vi "PeriodicTaskMatrix.vi"(8 "Error In":errorcluster, 9 "Smart Write (T)?":bool=TRUE, 10 "LEDs to Light":bool[][](array[boolean])=[[TRUE, TRUE, TRUE, TRUE, TRUE, TRUE, TRUE, FALSE], [TRUE, TRUE, TRUE, TRUE, TRUE, TRUE, FALSE, FALSE], [TRUE, TRUE, TRUE, TRUE, TRUE, FALSE, FALSE, FALSE], [TRUE, TRUE, TRUE, TRUE, FALSE, FALSE, FALSE, FALSE], [TRUE, TRUE, TRUE, FALSE, FALSE, FALSE, FALSE, FALSE], [TRUE, TRUE, FALSE, FALSE, FALSE, FALSE, FALSE, FALSE], [TRUE, FALSE, FALSE, FALSE, FALSE, FALSE, FALSE, FALSE], [FALSE, FALSE, FALSE, FALSE, FALSE, FALSE, FALSE, TRUE]], 11 "LINX Resource":T1) -> (0 "Error Out":errorcluster, 2 "Response":u8[](array[numeric]), 3 "LINX Resource":T1)   [LabVIEW 2014, in "LMH-LINX.lvlib" / "Interaction Parts Kit.lvlib"]
doc: "Updates the design shown on the LED matrix"
uses:
  <vilib>/MakerHub/LINX/Public/Sensors/Digilent/Interaction Parts Kit/Interaction Parts Kit.lvlib
  <vilib>/MakerHub/LINX/Private/Type Defs/LINX Ref.ctl
  <vilib>/MakerHub/LINX/Private/Type Defs/Platform.ctl
  <vilib>/MakerHub/LINX/Private/Type Defs/Interface.ctl
  <vilib>/MakerHub/LINX/Private/Device/Type Defs/LINX Device Config.ctl
  <vilib>/MakerHub/LINX/Private/Device/Type Defs/TCP Config.ctl
  <vilib>/MakerHub/LINX/Private/Device/Type Defs/Channels.ctl
  <vilib>/MakerHub/LINX/LMH-LINX.lvlib
  <vilib>/MakerHub/LINX/Private/Device/Device.lvlib
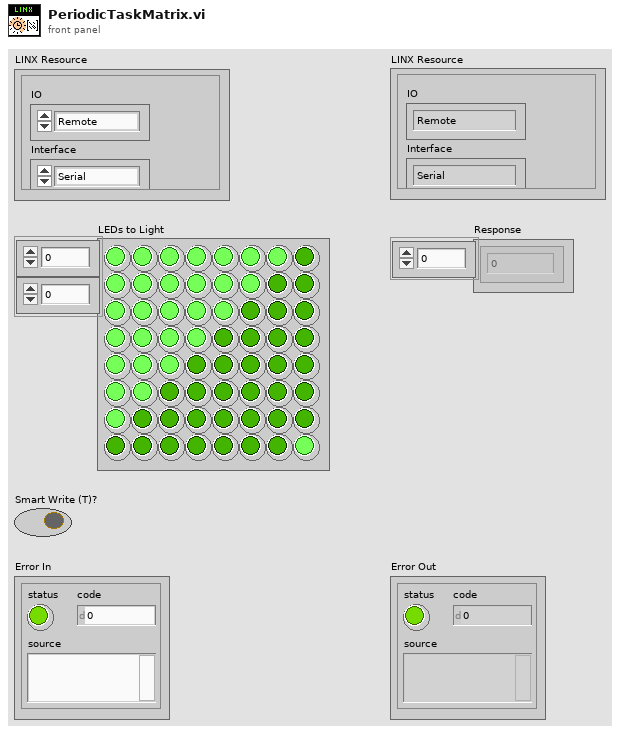
[diagram p1: front panel]
types:
  T1 = typedef "LMH-LINX.lvlib/LINX Ref.ctl" = cluster{"IO":T2, "Interface":T3, "LINX Device Config":T4}
  T2 = typedef "LMH-LINX.lvlib/Platform.ctl" = enum16{"Remote", "Local"}
  T3 = typedef "LMH-LINX.lvlib/Interface.ctl" = enum16{"Serial", "TCP"}
  T4 = typedef "LMH-LINX.lvlib/Device.lvlib/LINX Device Config.ctl" = cluster{"Interface":T3, "COM Port":refnum<visa-resource-name>, "TCP Configuration":T5, "Device Family":u8, "Device ID":u8, "Device Name":string, "TCP Ref":refnum<k5>, "Channels":T6}
  T5 = typedef "LMH-LINX.lvlib/Device.lvlib/TCP Config.ctl" = cluster{"IP Address":string, "Port":u16}
  T6 = typedef "LMH-LINX.lvlib/Channels.ctl" = cluster{"DI":u8[], "DO":u8[], "AI":u8[], "AO":u8[], "PWM":u8[], "QE":u8[], "UART":u8[], "I2C 2":u8[], "SPI":u8[], "CAN":u8[], "Servo":u8[], "AI Ref (V)":dbl, "AI Resolution (Bits)":u8, "AO Ref (V)":dbl, "AO Resolution (Bits)":u8}
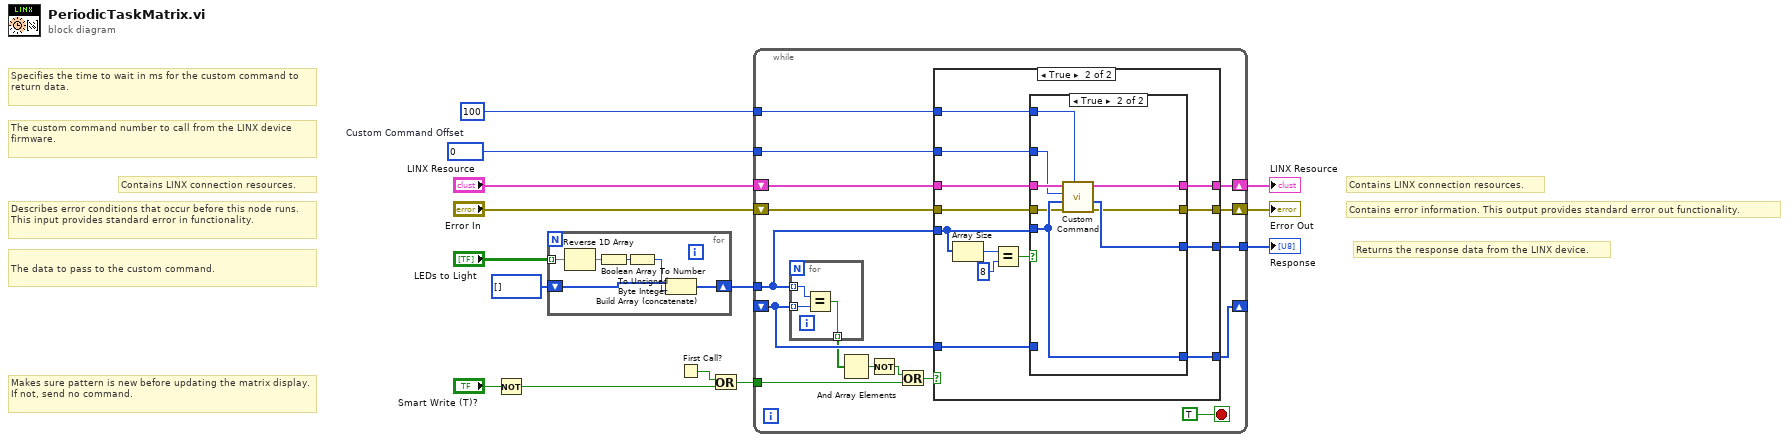
[diagram p0: block diagram]
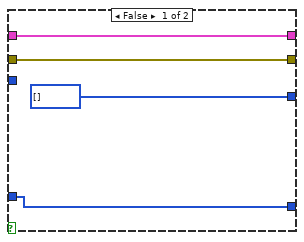
[diagram p2: hidden frame]
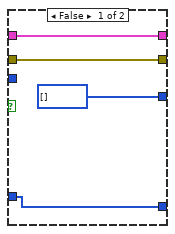
[diagram p3: hidden frame]
diagram:
  w7 = u16 0  # Custom Command Offset
  # "Makes sure pattern is new before updating the matrix display.  If not, send no command."
  # "The data to pass to the custom command."
  # "Specifies the time to wait in ms for the custom command to return data."
  # "The custom command number to call from the LINX device firmware."
  # "Returns the response data from the LINX device."
  # "Contains LINX connection resources."
  # "Contains error information. This output provides standard error out functionality."
  # "Contains LINX connection resources."
  # "Describes error conditions that occur before this node runs. This input provides standard error in functionality."
  n1 = Not(x="Smart Write (T)?") -> (.not. x?=w2:bool)
  n2 = for {
    tunnel: "LEDs to Light" -> [w20] mode=indexing
    shift-right: [w18] -> w5
    shift-left: u8[] [] -> [w17]
    n3 = Reverse 1D Array(array=w20) -> (reversed array=w19:bool[])
    n4 = Boolean Array To Number(Boolean array=w19) -> (number=w16:u32)
    n5 = To Unsigned Byte Integer(number=w16) -> (unsigned 8bit integer=w15:u8)
    n6 = Build Array (concatenate)(w17, w15) -> (w18:u8[])
  }
  n7 = First Call?() -> (First Call?: T/F=w4:bool)
  n8 = Or(x=w4, y=w2) -> (x .or. y?=w3:bool)
  n9 = while {
    tunnel: 100 ("Timeout (100 ms)") -> [w32]
    tunnel: w7 -> [w31]
    shift-right: [w33] -> w9
    shift-left: "LINX Resource" -> [w36]
    shift-right: [w34] -> w10
    shift-left: "Error In" -> [w35]
    shift-right: [w28] -> _
    shift-left: _ -> [w26]
    tunnel: [w29] -> w6
    tunnel: w5 -> [w27]
    tunnel: w3 -> [w21]
    stop <- TRUE stop-if-true
    n10 = for {
      tunnel: w27 -> [w68] mode=indexing
      tunnel: w26 -> [w67] mode=indexing
      tunnel: [w66] -> w25 mode=indexing
      n11 = Equal?(x=w68, y=w67) -> (x = y?=w66:bool)
    }
    n12 = And Array Elements(Boolean array=w25) -> (logical AND=w24:bool)
    n13 = Not(x=w24) -> (.not. x?=w23:bool)
    n14 = Or(x=w23, y=w21) -> (x .or. y?=w22:bool)
    n15 = case shown="True" w22 {
      tunnel: w36 -> [w40 w53]
      tunnel: w35 -> [w38 w52]
      tunnel: [w38 w51] -> w34
      tunnel: [w40 w50] -> w33
      tunnel: w32 -> [_ w49]
      tunnel: w31 -> [_ w48]
      tunnel: [u8[] [] ("Response") w44] -> w29
      tunnel: w27 -> [_ w43]
      tunnel: [w37 w42] -> w28
      tunnel: w26 -> [w37 w41]
      frame False {
      }
      frame True {
        n16 = Array Size(array=w43) -> (size(s)=w47:i32)
        n17 = Equal?(x=w47, y=8) -> (x = y?=w45:bool)
        n18 = case shown="True" w45 {
          tunnel: w53 -> [w56 w65]
          tunnel: w52 -> [w55 w61]
          tunnel: [w55 w58] -> w51
          tunnel: [w56 w60] -> w50
          tunnel: [u8[] [] ("Response") w59] -> w44
          tunnel: w49 -> [_ w64]
          tunnel: w48 -> [_ w63]
          tunnel: w43 -> [_ w62]
          tunnel: [w57 w62] -> w42
          tunnel: w41 -> [w57 _]
          frame False {
          }
          frame True {
            n19 = call <vilib>:"Custom Command.vi"("Timeout (100 ms)"=w64, "Error In"=w61, "Data"=w62, "Custom Command Number"=w63, "LINX Resource"=w65) -> ("Error Out"=w58:errorcluster, "Response"=w59:u8[], "LINX Resource"=w60:T1)  [unwired: 3 in, 1 out]
          }
        }
      }
    }
  }
  "Error Out" <- w10
  "LINX Resource" <- w9
  "Response" <- w6
